vi "Set SPAN Component Daten aufzeichnen.vi"(10 "Daten aufzeichnen":T1, 11 "Daten aufzeichnen Offset Cluster":T2) -> ()   [LabVIEW 2020, in "Linearisierung v2.lvlib" / "SpanEinstellungen.lvlib"]
uses:
  SpanEinstellungen.lvlib
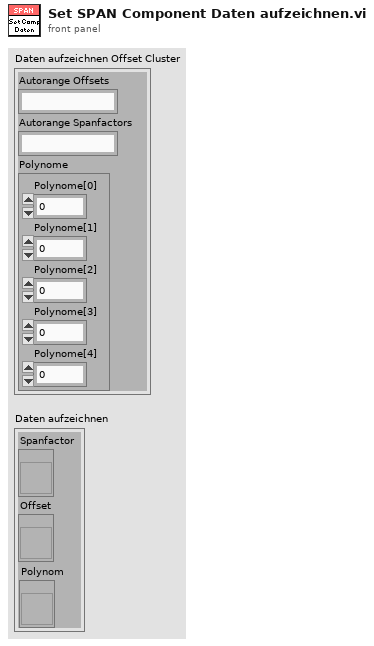
[diagram p1: front panel]
types:
  T1 = cluster{"Spanfactor":refnum<vi>, "Offset":refnum<vi>, "Polynom":refnum<vi>}
  T2 = cluster{"Autorange Offsets":string, "Autorange Spanfactors":string, "Polynome":cluster{"Polynome[0]":dbl, "Polynome[1]":dbl, "Polynome[2]":dbl, "Polynome[3]":dbl, "Polynome[4]":dbl}}
  T3 = cluster{"Polynome[0]":dbl, "Polynome[1]":dbl, "Polynome[2]":dbl, "Polynome[3]":dbl, "Polynome[4]":dbl}
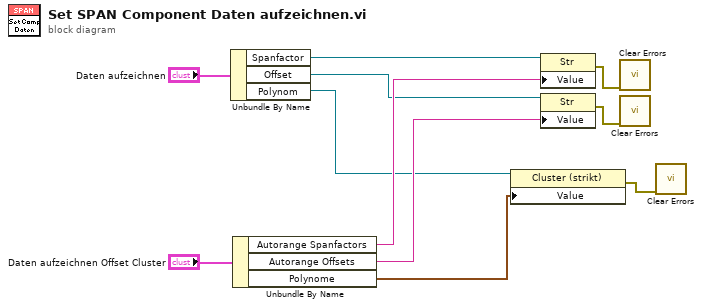
[diagram p0: block diagram]
diagram:
  n1 = Unbundle By Name("Daten aufzeichnen") -> ("Spanfactor"=w10:refnum<vi>, "Offset"=w8:refnum<vi>, "Polynom"=w2:refnum<vi>)
  n2 = Unbundle By Name("Daten aufzeichnen Offset Cluster") -> ("Autorange Spanfactors"=w9:string, "Autorange Offsets"=w7:string, "Polynome"=w1:T3)
  n3 = property class="Cluster (strikt)"(reference=w2, "Value"=w1) -> (error out=w3:errorcluster)  [unwired: 1 in, 1 out]
  n4 = property class="Str"(reference=w10, "Value"=w9) -> (error out=w6:errorcluster)  [unwired: 1 in, 1 out]
  n5 = property class="Str"(reference=w8, "Value"=w7) -> (error out=w5:errorcluster)  [unwired: 1 in, 1 out]
  n6 = call <vilib>:"Clear Errors.vi"("error in (no error)"=w6) -> ()  [unwired: 5 in, 2 out]
  n7 = call <vilib>:"Clear Errors.vi"("error in (no error)"=w5) -> ()  [unwired: 5 in, 2 out]
  n8 = call <vilib>:"Clear Errors.vi"("error in (no error)"=w3) -> ()  [unwired: 5 in, 2 out]
